vi "RtdeWriteInputs.vi"(8 "Data":T1, 10 "Rtde":refnum<k24>, 11 "error in":errorcluster) -> (3 "error out":errorcluster)   [LabVIEW 2023, in "UnderAutomation.UniversalRobots.lvlib"]
uses:
  UnderAutomation.UniversalRobots.lvlib
  C:/Users/fg/Documents/UniversalRobots.vi/UnderAutomation.UniversalRobots/lib/UnderAutomation.UniversalRobots.dll
  lib/UnderAutomation.UniversalRobots.dll
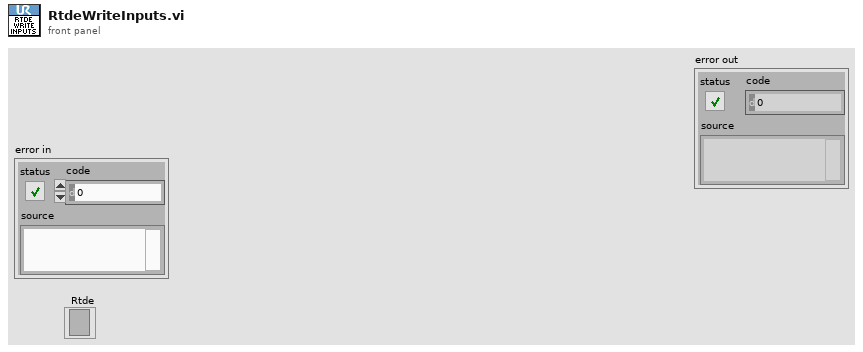
[diagram p1: front panel]
types:
  T1 = cluster{"ConfigurableDigitalOutput":u8, "ConfigurableDigitalOutputMask":u8, "ExternalForceTorque":cluster{"X":dbl, "Y":dbl, "Z":dbl, "Rx":dbl, "Ry":dbl, "Rz":dbl}, "InputBitRegisters":cluster{"X64":bool, "X65":bool, "X66":bool, "X67":bool, "X68":bool, "X69":bool, "X70":bool, "X71":bool, "X72":bool, "X73":bool, "X74":bool, "X75":bool, "X76":bool, "X77":bool, "X78":bool, "X79":bool, "X80":bool, "X81":bool, "X82":bool, "X83":bool, "X84":bool, "X85":bool, "X86":bool, "X87":bool, "X88":bool, "X89":bool, "X90":bool, "X91":bool, "X92":bool, "X93":bool, "X94":bool, "X95":bool, "X96":bool, "X97":bool, "X98":bool, "X99":bool, "X100":bool, "X101":bool, "X102":bool, "X103":bool, "X104":bool, "X105":bool, "X106":bool, "X107":bool, "X108":bool, "X109":bool, "X110":bool, "X111":bool, "X112":bool, "X113":bool, "X114":bool, "X115":bool, "X116":bool, "X117":bool, "X118":bool, "X119":bool, "X120":bool, "X121":bool, "X122":bool, "X123":bool, "X124":bool, "X125":bool, "X126":bool, "X127":bool}, "InputBtRegisters0To31":u32, "InputBtRegisters32To63":u32, "InputDoubleRegisters":cluster{"X0":dbl, "X1":dbl, "X2":dbl, "X3":dbl, "X4":dbl, "X5":dbl, "X6":dbl, "X7":dbl, "X8":dbl, "X9":dbl, "X10":dbl, "X11":dbl, "X12":dbl, "X13":dbl, "X14":dbl, "X15":dbl, "X16":dbl, "X17":dbl, "X18":dbl, "X19":dbl, "X20":dbl, "X21":dbl, "X22":dbl, "X23":dbl, "X24":dbl, "X25":dbl, "X26":dbl, "X27":dbl, "X28":dbl, "X29":dbl, "X30":dbl, "X31":dbl, "X32":dbl, "X33":dbl, "X34":dbl, "X35":dbl, "X36":dbl, "X37":dbl, "X38":dbl, "X39":dbl, "X40":dbl, "X41":dbl, "X42":dbl, "X43":dbl, "X44":dbl, "X45":dbl, "X46":dbl, "X47":dbl}, "InputIntRegisters":cluster{"X0":i32, "X1":i32, "X2":i32, "X3":i32, "X4":i32, "X5":i32, "X6":i32, "X7":i32, "X8":i32, "X9":i32, "X10":i32, "X11":i32, "X12":i32, "X13":i32, "X14":i32, "X15":i32, "X16":i32, "X17":i32, "X18":i32, "X19":i32, "X20":i32, "X21":i32, "X22":i32, "X23":i32, "X24":i32, "X25":i32, "X26":i32, "X27":i32, "X28":i32, "X29":i32, "X30":i32, "X31":i32, "X32":i32, "X33":i32, "X34":i32, "X35":i32, "X36":i32, "X37":i32, "X38":i32, "X39":i32, "X40":i32, "X41":i32, "X42":i32, "X43":i32, "X44":i32, "X45":i32, "X46":i32, "X47":i32}, "SpeedSliderFraction":dbl, "SpeedSliderMask":u32, "StandardAnalogOutput0":dbl, "StandardAnalogOutput1":dbl, "StandardAnalogOutputMask":u8, "StandardAnalogOutputType":u8, "StandardDigitalOutput":u8, "StandardDigitalOutputMask":u8}
  T2 = cluster{"X":dbl, "Y":dbl, "Z":dbl, "Rx":dbl, "Ry":dbl, "Rz":dbl}
  T3 = cluster{"X64":bool, "X65":bool, "X66":bool, "X67":bool, "X68":bool, "X69":bool, "X70":bool, "X71":bool, "X72":bool, "X73":bool, "X74":bool, "X75":bool, "X76":bool, "X77":bool, "X78":bool, "X79":bool, "X80":bool, "X81":bool, "X82":bool, "X83":bool, "X84":bool, "X85":bool, "X86":bool, "X87":bool, "X88":bool, "X89":bool, "X90":bool, "X91":bool, "X92":bool, "X93":bool, "X94":bool, "X95":bool, "X96":bool, "X97":bool, "X98":bool, "X99":bool, "X100":bool, "X101":bool, "X102":bool, "X103":bool, "X104":bool, "X105":bool, "X106":bool, "X107":bool, "X108":bool, "X109":bool, "X110":bool, "X111":bool, "X112":bool, "X113":bool, "X114":bool, "X115":bool, "X116":bool, "X117":bool, "X118":bool, "X119":bool, "X120":bool, "X121":bool, "X122":bool, "X123":bool, "X124":bool, "X125":bool, "X126":bool, "X127":bool}
  T4 = cluster{"X0":dbl, "X1":dbl, "X2":dbl, "X3":dbl, "X4":dbl, "X5":dbl, "X6":dbl, "X7":dbl, "X8":dbl, "X9":dbl, "X10":dbl, "X11":dbl, "X12":dbl, "X13":dbl, "X14":dbl, "X15":dbl, "X16":dbl, "X17":dbl, "X18":dbl, "X19":dbl, "X20":dbl, "X21":dbl, "X22":dbl, "X23":dbl, "X24":dbl, "X25":dbl, "X26":dbl, "X27":dbl, "X28":dbl, "X29":dbl, "X30":dbl, "X31":dbl, "X32":dbl, "X33":dbl, "X34":dbl, "X35":dbl, "X36":dbl, "X37":dbl, "X38":dbl, "X39":dbl, "X40":dbl, "X41":dbl, "X42":dbl, "X43":dbl, "X44":dbl, "X45":dbl, "X46":dbl, "X47":dbl}
  T5 = cluster{"X0":i32, "X1":i32, "X2":i32, "X3":i32, "X4":i32, "X5":i32, "X6":i32, "X7":i32, "X8":i32, "X9":i32, "X10":i32, "X11":i32, "X12":i32, "X13":i32, "X14":i32, "X15":i32, "X16":i32, "X17":i32, "X18":i32, "X19":i32, "X20":i32, "X21":i32, "X22":i32, "X23":i32, "X24":i32, "X25":i32, "X26":i32, "X27":i32, "X28":i32, "X29":i32, "X30":i32, "X31":i32, "X32":i32, "X33":i32, "X34":i32, "X35":i32, "X36":i32, "X37":i32, "X38":i32, "X39":i32, "X40":i32, "X41":i32, "X42":i32, "X43":i32, "X44":i32, "X45":i32, "X46":i32, "X47":i32}
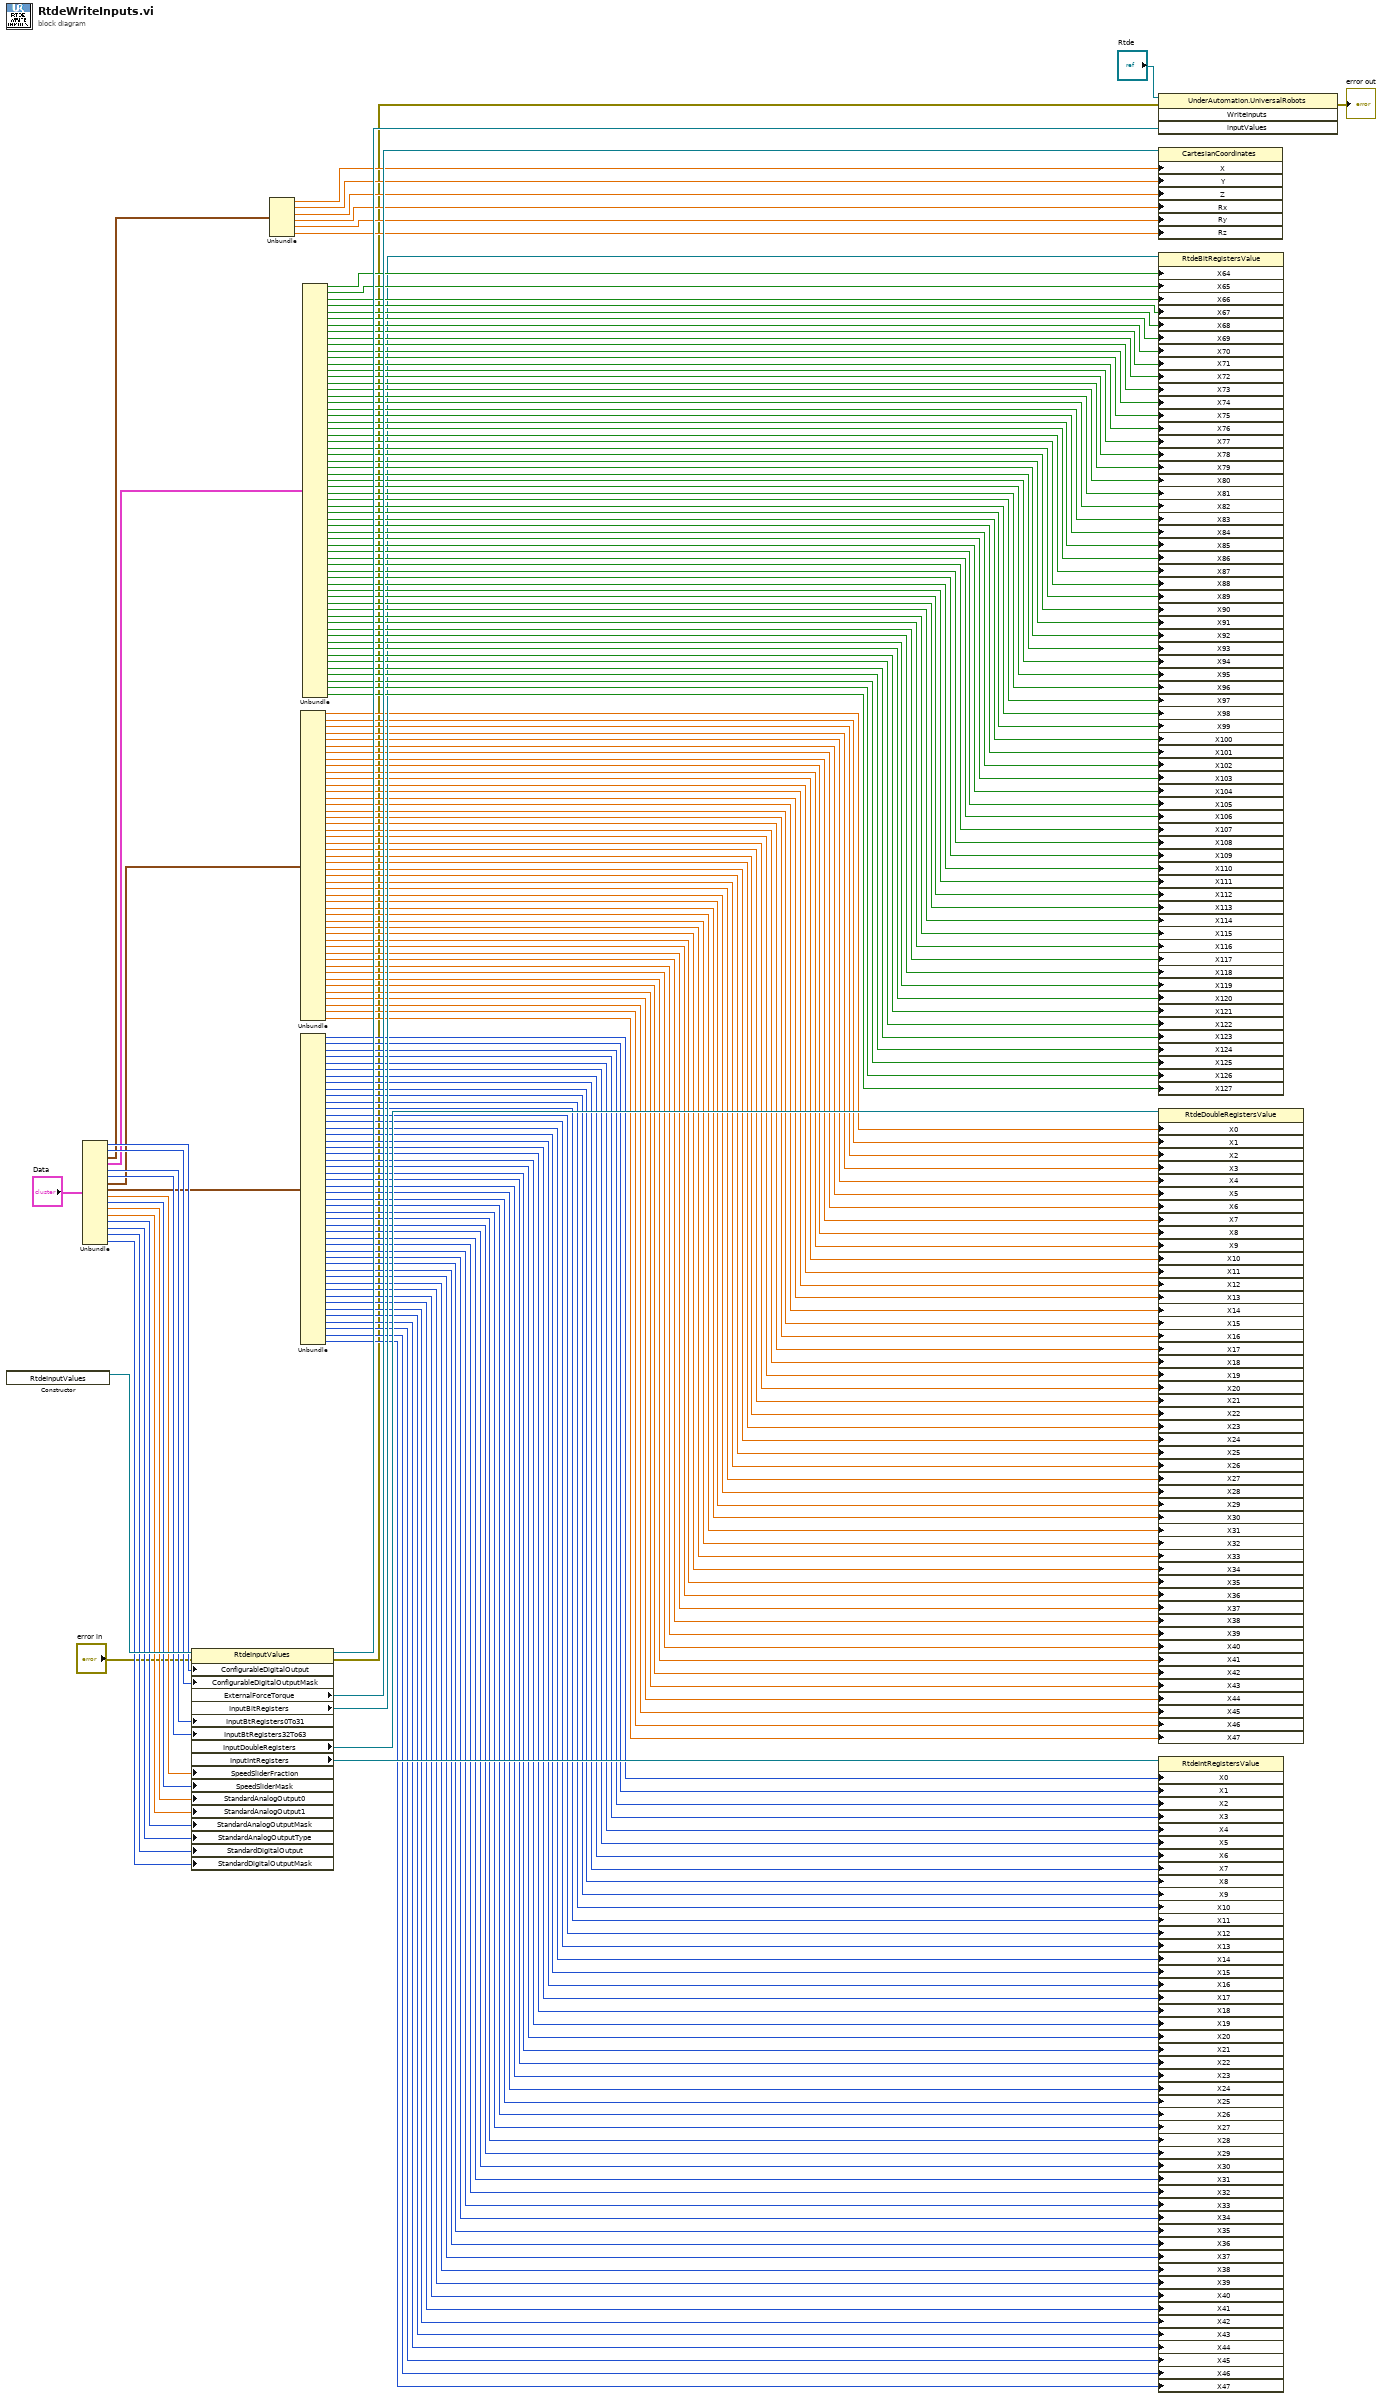
[diagram p0: block diagram]
diagram:
  n1 = constructor class="RtdeInputValues"() -> (reference out=w192:refnum<k24>)  [unwired: 3 in, 2 out]
  n2 = Unbundle("Data") -> ("ConfigurableDigitalOutput"=w188:u8, "ConfigurableDigitalOutputMask"=w187:u8, "ExternalForceTorque"=w176:T2, "InputBitRegisters"=w168:T3, "InputBtRegisters0To31"=w186:u32, "InputBtRegisters32To63"=w185:u32, "InputDoubleRegisters"=w103:T4, "InputIntRegisters"=w51:T5, "SpeedSliderFraction"=w184:dbl, "SpeedSliderMask"=w183:u32, "StandardAnalogOutput0"=w182:dbl, "StandardAnalogOutput1"=w181:dbl, "StandardAnalogOutputMask"=w180:u8, "StandardAnalogOutputType"=w179:u8, "StandardDigitalOutput"=w178:u8, "StandardDigitalOutputMask"=w177:u8)
  n3 = property class="RtdeInputValues"(reference=w192, error in="error in", "ConfigurableDigitalOutput"=w188, "ConfigurableDigitalOutputMask"=w187, "InputBtRegisters0To31"=w186, "InputBtRegisters32To63"=w185, "SpeedSliderFraction"=w184, "SpeedSliderMask"=w183, "StandardAnalogOutput0"=w182, "StandardAnalogOutput1"=w181, "StandardAnalogOutputMask"=w180, "StandardAnalogOutputType"=w179, "StandardDigitalOutput"=w178, "StandardDigitalOutputMask"=w177) -> (reference out=w191:refnum<k24>, error out=w1:errorcluster, "ExternalForceTorque"=w175:refnum<k24>, "InputBitRegisters"=w102:refnum<k24>, "InputDoubleRegisters"=w101:refnum<k24>, "InputIntRegisters"=w52:refnum<k24>)
  n4 = Unbundle(w176) -> ("X"=w174:dbl, "Y"=w173:dbl, "Z"=w171:dbl, "Rx"=w172:dbl, "Ry"=w170:dbl, "Rz"=w169:dbl)
  n5 = Unbundle(w103) -> ("X0"=w100:dbl, "X1"=w99:dbl, "X2"=w98:dbl, "X3"=w97:dbl, "X4"=w96:dbl, "X5"=w95:dbl, "X6"=w94:dbl, "X7"=w93:dbl, "X8"=w92:dbl, "X9"=w91:dbl, "X10"=w90:dbl, "X11"=w89:dbl, "X12"=w88:dbl, "X13"=w87:dbl, "X14"=w84:dbl, "X15"=w86:dbl, "X16"=w85:dbl, "X17"=w83:dbl, "X18"=w82:dbl, "X19"=w81:dbl, "X20"=w80:dbl, "X21"=w79:dbl, "X22"=w78:dbl, "X23"=w77:dbl, "X24"=w76:dbl, "X25"=w75:dbl, "X26"=w74:dbl, "X27"=w73:dbl, "X28"=w72:dbl, "X29"=w71:dbl, "X30"=w70:dbl, "X31"=w69:dbl, "X32"=w68:dbl, "X33"=w67:dbl, "X34"=w66:dbl, "X35"=w64:dbl, "X36"=w65:dbl, "X37"=w63:dbl, "X38"=w62:dbl, "X39"=w61:dbl, "X40"=w60:dbl, "X41"=w59:dbl, "X42"=w58:dbl, "X43"=w57:dbl, "X44"=w56:dbl, "X45"=w55:dbl, "X46"=w54:dbl, "X47"=w53:dbl)
  n6 = Unbundle(w51) -> ("X0"=w50:i32, "X1"=w49:i32, "X2"=w48:i32, "X3"=w47:i32, "X4"=w46:i32, "X5"=w45:i32, "X6"=w44:i32, "X7"=w43:i32, "X8"=w42:i32, "X9"=w41:i32, "X10"=w40:i32, "X11"=w39:i32, "X12"=w38:i32, "X13"=w37:i32, "X14"=w36:i32, "X15"=w35:i32, "X16"=w34:i32, "X17"=w33:i32, "X18"=w32:i32, "X19"=w31:i32, "X20"=w30:i32, "X21"=w29:i32, "X22"=w28:i32, "X23"=w27:i32, "X24"=w26:i32, "X25"=w25:i32, "X26"=w24:i32, "X27"=w23:i32, "X28"=w22:i32, "X29"=w21:i32, "X30"=w20:i32, "X31"=w19:i32, "X32"=w18:i32, "X33"=w17:i32, "X34"=w16:i32, "X35"=w15:i32, "X36"=w14:i32, "X37"=w13:i32, "X38"=w11:i32, "X39"=w12:i32, "X40"=w10:i32, "X41"=w9:i32, "X42"=w8:i32, "X43"=w7:i32, "X44"=w6:i32, "X45"=w5:i32, "X46"=w4:i32, "X47"=w3:i32)
  n7 = Unbundle(w168) -> ("X64"=w167:bool, "X65"=w166:bool, "X66"=w165:bool, "X67"=w164:bool, "X68"=w163:bool, "X69"=w162:bool, "X70"=w161:bool, "X71"=w160:bool, "X72"=w159:bool, "X73"=w158:bool, "X74"=w157:bool, "X75"=w156:bool, "X76"=w155:bool, "X77"=w154:bool, "X78"=w153:bool, "X79"=w152:bool, "X80"=w151:bool, "X81"=w150:bool, "X82"=w149:bool, "X83"=w148:bool, "X84"=w147:bool, "X85"=w146:bool, "X86"=w145:bool, "X87"=w144:bool, "X88"=w143:bool, "X89"=w142:bool, "X90"=w141:bool, "X91"=w140:bool, "X92"=w139:bool, "X93"=w138:bool, "X94"=w137:bool, "X95"=w136:bool, "X96"=w135:bool, "X97"=w134:bool, "X98"=w133:bool, "X99"=w132:bool, "X100"=w131:bool, "X101"=w130:bool, "X102"=w129:bool, "X103"=w128:bool, "X104"=w127:bool, "X105"=w126:bool, "X106"=w125:bool, "X107"=w124:bool, "X108"=w123:bool, "X109"=w122:bool, "X110"=w121:bool, "X111"=w120:bool, "X112"=w119:bool, "X113"=w118:bool, "X114"=w117:bool, "X115"=w116:bool, "X116"=w115:bool, "X117"=w114:bool, "X118"=w112:bool, "X119"=w113:bool, "X120"=w111:bool, "X121"=w110:bool, "X122"=w109:bool, "X123"=w108:bool, "X124"=w107:bool, "X125"=w106:bool, "X126"=w105:bool, "X127"=w104:bool)
  n8 = invoke class="UnderAutomation.UniversalRobots" method="WriteInputs"(reference="Rtde", error in=w1, "inputValues"=w191) -> (error out=→"error out":errorcluster)  [unwired: 1 in, 3 out]
  n9 = property class="CartesianCoordinates"(reference=w175, "X"=w174, "Y"=w173, "Z"=w171, "Rx"=w172, "Ry"=w170, "Rz"=w169) -> ()  [unwired: 1 in, 2 out]
  n10 = property class="RtdeBitRegistersValue"(reference=w102, "X64"=w167, "X65"=w166, "X66"=w165, "X67"=w164, "X68"=w163, "X69"=w162, "X70"=w161, "X71"=w160, "X72"=w159, "X73"=w158, "X74"=w157, "X75"=w156, "X76"=w155, "X77"=w154, "X78"=w153, "X79"=w152, "X80"=w151, "X81"=w150, "X82"=w149, "X83"=w148, "X84"=w147, "X85"=w146, "X86"=w145, "X87"=w144, "X88"=w143, "X89"=w142, "X90"=w141, "X91"=w140, "X92"=w139, "X93"=w138, "X94"=w137, "X95"=w136, "X96"=w135, "X97"=w134, "X98"=w133, "X99"=w132, "X100"=w131, "X101"=w130, "X102"=w129, "X103"=w128, "X104"=w127, "X105"=w126, "X106"=w125, "X107"=w124, "X108"=w123, "X109"=w122, "X110"=w121, "X111"=w120, "X112"=w119, "X113"=w118, "X114"=w117, "X115"=w116, "X116"=w115, "X117"=w114, "X118"=w112, "X119"=w113, "X120"=w111, "X121"=w110, "X122"=w109, "X123"=w108, "X124"=w107, "X125"=w106, "X126"=w105, "X127"=w104) -> ()  [unwired: 1 in, 2 out]
  n11 = property class="RtdeDoubleRegistersValue"(reference=w101, "X0"=w100, "X1"=w99, "X2"=w98, "X3"=w97, "X4"=w96, "X5"=w95, "X6"=w94, "X7"=w93, "X8"=w92, "X9"=w91, "X10"=w90, "X11"=w89, "X12"=w88, "X13"=w87, "X14"=w84, "X15"=w86, "X16"=w85, "X17"=w83, "X18"=w82, "X19"=w81, "X20"=w80, "X21"=w79, "X22"=w78, "X23"=w77, "X24"=w76, "X25"=w75, "X26"=w74, "X27"=w73, "X28"=w72, "X29"=w71, "X30"=w70, "X31"=w69, "X32"=w68, "X33"=w67, "X34"=w66, "X35"=w64, "X36"=w65, "X37"=w63, "X38"=w62, "X39"=w61, "X40"=w60, "X41"=w59, "X42"=w58, "X43"=w57, "X44"=w56, "X45"=w55, "X46"=w54, "X47"=w53) -> ()  [unwired: 1 in, 2 out]
  n12 = property class="RtdeIntRegistersValue"(reference=w52, "X0"=w50, "X1"=w49, "X2"=w48, "X3"=w47, "X4"=w46, "X5"=w45, "X6"=w44, "X7"=w43, "X8"=w42, "X9"=w41, "X10"=w40, "X11"=w39, "X12"=w38, "X13"=w37, "X14"=w36, "X15"=w35, "X16"=w34, "X17"=w33, "X18"=w32, "X19"=w31, "X20"=w30, "X21"=w29, "X22"=w28, "X23"=w27, "X24"=w26, "X25"=w25, "X26"=w24, "X27"=w23, "X28"=w22, "X29"=w21, "X30"=w20, "X31"=w19, "X32"=w18, "X33"=w17, "X34"=w16, "X35"=w15, "X36"=w14, "X37"=w13, "X38"=w11, "X39"=w12, "X40"=w10, "X41"=w9, "X42"=w8, "X43"=w7, "X44"=w6, "X45"=w5, "X46"=w4, "X47"=w3) -> ()  [unwired: 1 in, 2 out]
